vi "Update User Input Control.vi"(8 "error in (no error)":errorcluster, 10 "ATM State":T1, 11 "ATM View Model in":refnum<class "ATM View Model.lvclass">) -> (0 "error out":errorcluster)   [LabVIEW 2020, in "ATM View Model.lvclass"]
uses:
  ATM View Model.lvclass
  ATM Controller/State.ctl
  Controls.ctl
  ATM View Model.lvclass/ATM View Model.ctl
  ATM Controller/ATM Controller.lvclass
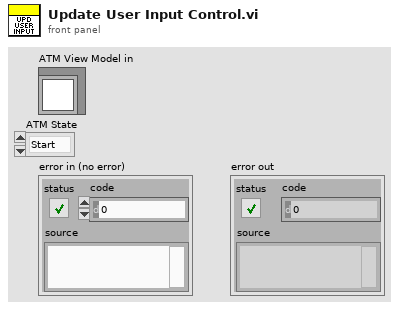
[diagram p1: front panel]
types:
  T1 = typedef "ATM Controller.lvclass/State.ctl" = enum16{"Start", "Card Inserted", "Verification Failed", "Verification Succeeded", "Depositing", "Depositing Completed", "Terminate"}
  T2 = typedef "ATM View Model.lvclass/Controls.ctl" = enum16{"User Input", "Enter", "Left Menu", "Right Menu", "Left Button", "Right Button", "Card Simulator"}
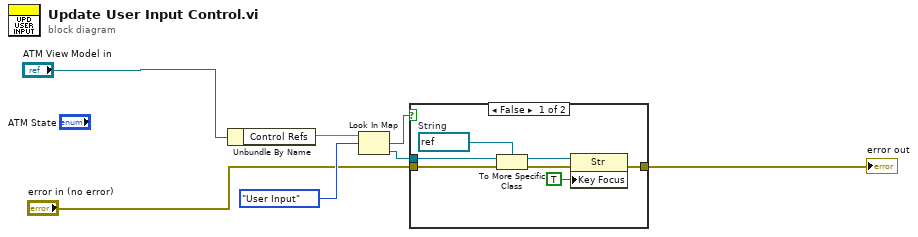
[diagram p0: block diagram]
diagram:
  n1 = Unbundle By Name("ATM View Model in") -> ("Control Refs"=w3:map{T2, refnum<vi>})
  n2 = Look In Map(map=w3, key=Controls."User Input") -> (key not found?=w7:bool, value=w5:refnum<vi>)  [unwired: 1 in]
  n3 = case shown="False" w7 {
    tunnel: "error in (no error)" -> [w14 w15]
    tunnel: w5 -> [w12 _]
    tunnel: [w10 w15] -> w6
    frame False {
      w11 = refnum<vi> refnum  # String
      n4 = To More Specific Class(target class=w11, reference=w12, error in=w14) -> (specific class reference=w9:refnum<vi>, error out=w13:errorcluster)
      n5 = property class="Str"(reference=w9, error in=w13, "Key Focus"=TRUE) -> (error out=w10:errorcluster)  [unwired: 1 out]
    }
    frame True {
    }
  }
  "error out" <- w6
